vi "GPS-1仪器串口通讯.vi"(0 "VISA resource name":refnum<visa-resource-name>="COM3", 4 "baud rate (9600)":u32=9600, 7 "错误常量 2":errorcluster caption="错误常量") -> (11 "错误常量":errorcluster, 12 "速率":string, 13 "经度":string, 14 "定位信息":string, 15 "UTC日期":string, 17 "航向":string, 18 "UTC时间":string, 19 "纬度":string)   [LabVIEW 2016]
uses:
  <vilib>/Instr/_visa.llb/VISA Configure Serial Port (Instr).vi
panel:
  out "数组":string[](array[string])
  out "字符串 3":string
  out "长度 2":i32
  in  "字符串 2":string
  out "长度":i32
  in  "字符串":string
  out "返回数 2":u32
  out "read buffer":string
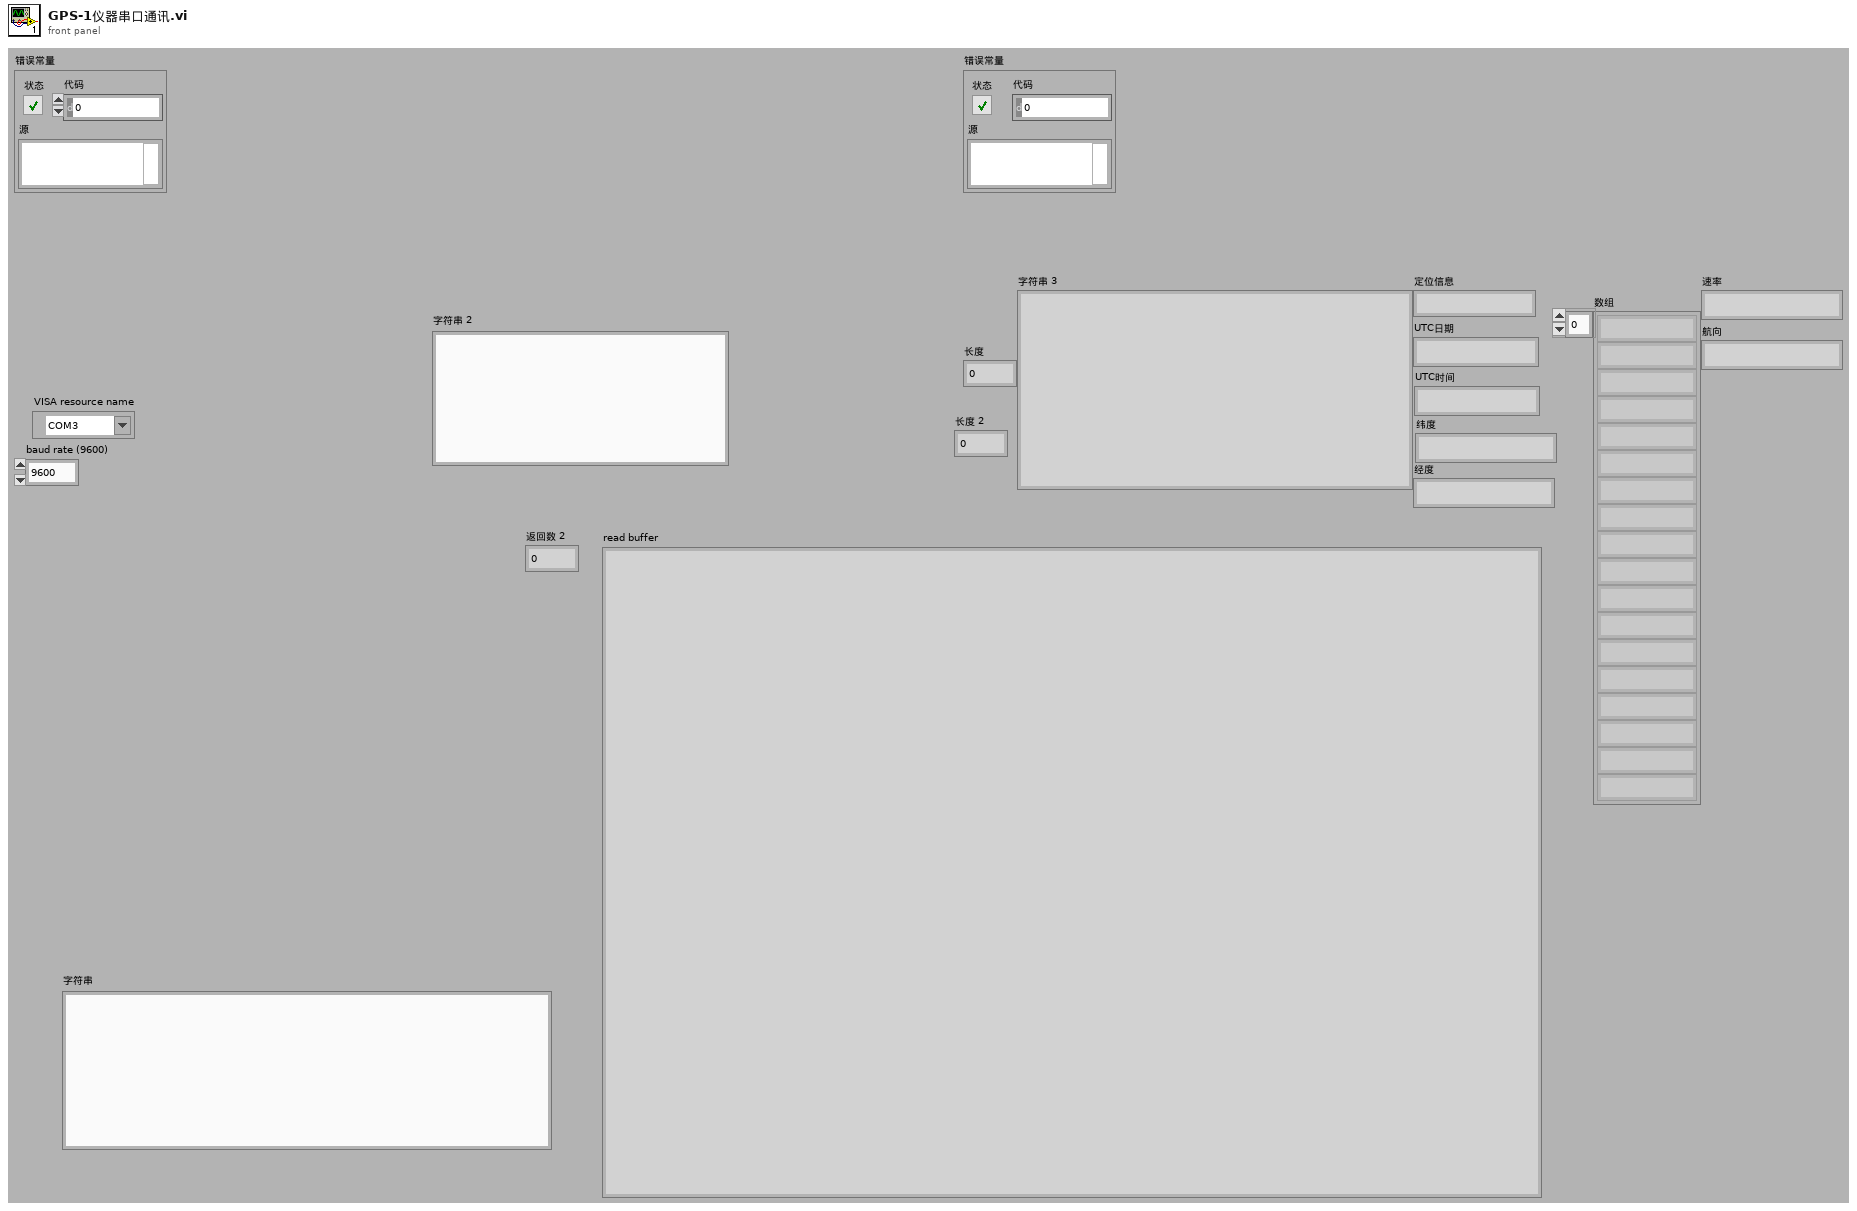
[diagram p1: front panel]
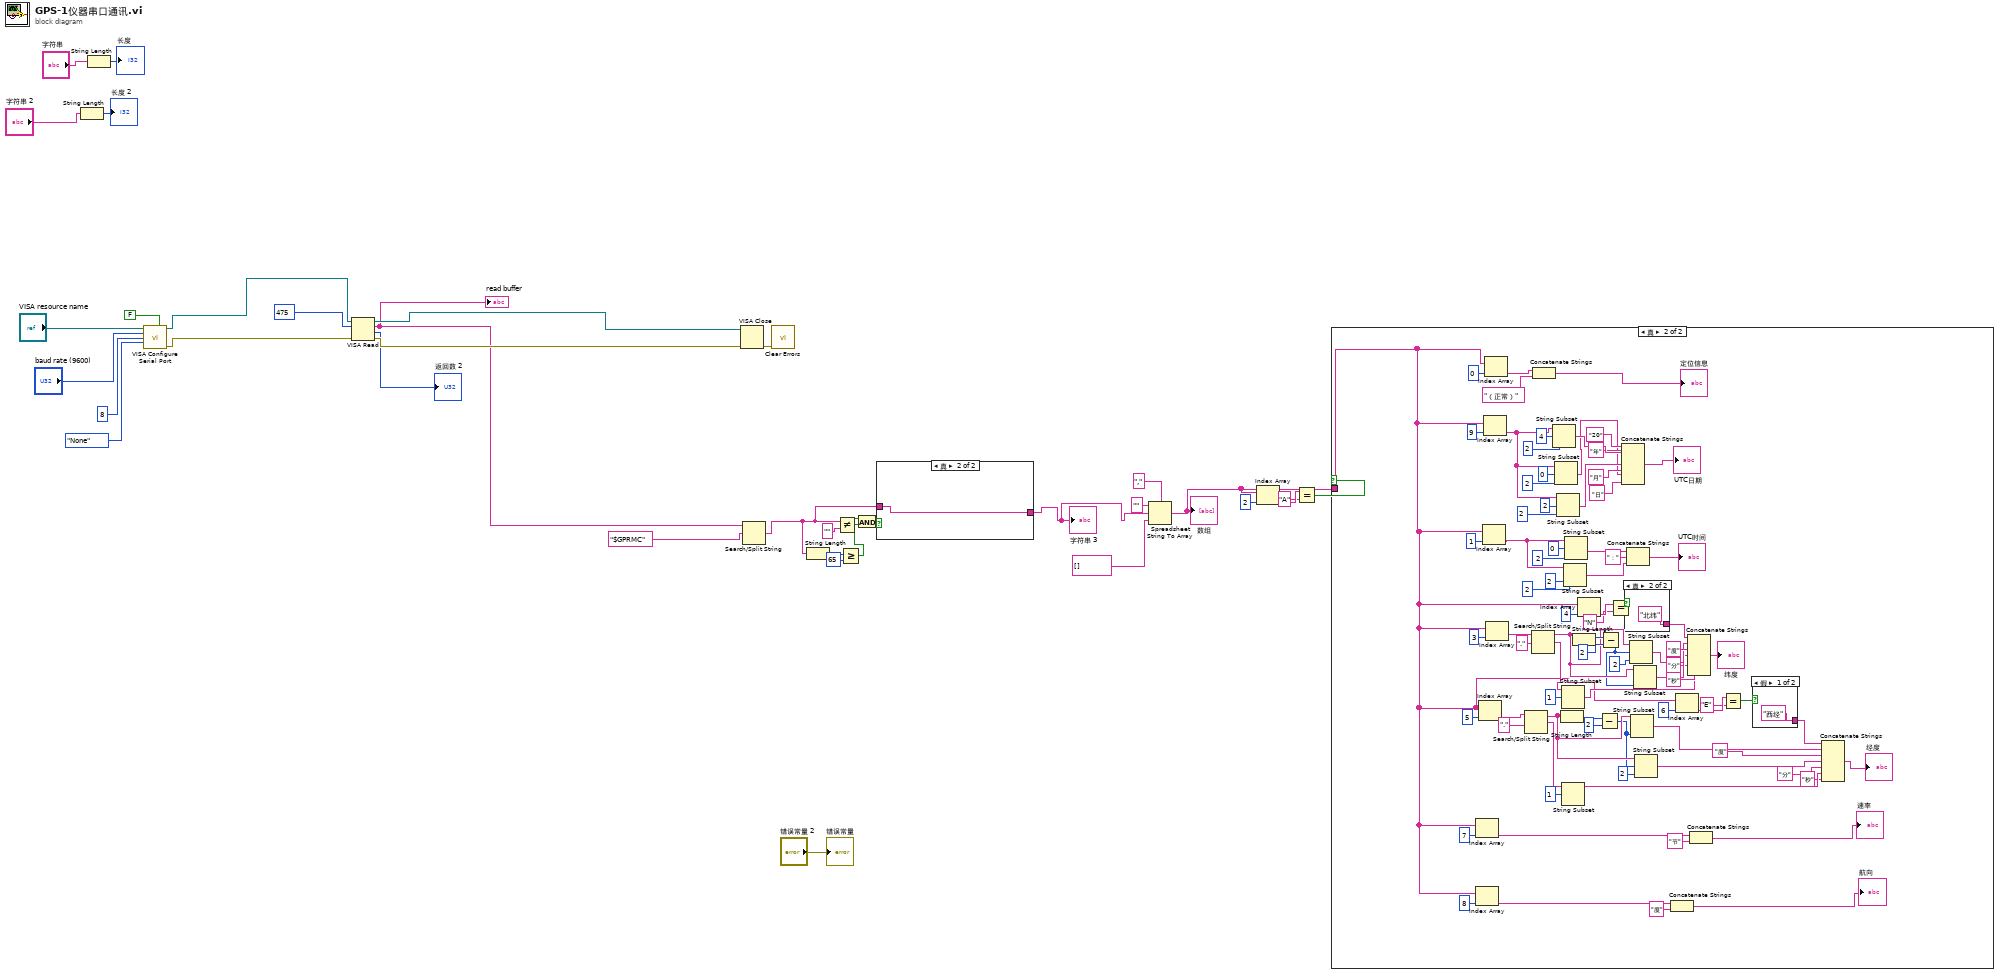
[diagram p0: block diagram]
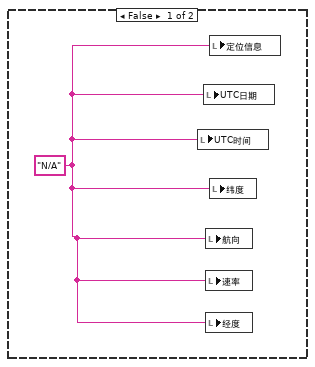
[diagram p2: hidden frame]
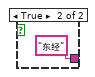
[diagram p3: hidden frame]
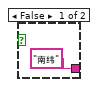
[diagram p4: hidden frame]
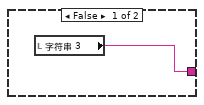
[diagram p5: hidden frame]
diagram:
  n1 = String Length(string="字符串 2") -> (length=→"长度 2":i32)
  n2 = String Length(string="字符串") -> (length=→"长度":i32)
  n3 = call-poly "VISA Configure Serial Port"("VISA resource name"="VISA resource name", "Enable Termination\nChar (T)"=FALSE ("Enable Termination\nChar (T)"), "baud rate (9600)"="baud rate (9600)", "data bits (8)"=u16 8, "parity (0:none)"=enum16{"None", "Odd", "Even", "Mark", "Space"}."None") -> ("VISA resource name out"=w23:refnum<visa-resource-name>, "error out"=w27:errorcluster)  [unwired: 9 in]
  n4 = VISA Read(VISA resource name=w23, byte count=u32 475 ("字节总数"), error in (no error)=w27) -> (VISA resource name out=w26:refnum<visa-resource-name>, read buffer=w19:string, return count=→"返回数 2":u32, error out=w32:errorcluster)
  "read buffer" <- w19
  n5 = VISA Close(VISA resource name=w26, error in (no error)=w32) -> (error out=w29:errorcluster)
  n6 = Search/Split String(string=w19, search string/char (-)="$GPRMC" ("搜索字符串/字符(-)")) -> (match + rest of string=w13:string)  [unwired: 1 in, 2 out]
  n7 = call <vilib>:"Clear Errors.vi"("error in (no error)"=w29) -> ()  [unwired: 5 in, 2 out]
  n8 = String Length(string=w13) -> (length=w14:i32)
  n9 = Not Equal?(x=w13, y="") -> (x != y?=w16:bool)
  n10 = Greater Or Equal?(x=w14, y=65) -> (x >= y?=w11:bool)
  n11 = And(x=w11, y=w16) -> (x .and. y?=w15:bool)
  n12 = case shown="真" w15 {
    tunnel: w13 -> [_ w37]
    tunnel: [w36 w37] -> w10
    frame False {
      n13 = local read "字符串 3"() -> (w36:string)
    }
    frame True {
    }
  }
  "字符串 3" <- w10
  n14 = Spreadsheet String To Array(delimiter (Tab)="," ("分隔符(Tab)"), format string="" ("格式字符串"), spreadsheet string=w10, array type (2D Dbl)=string[] []) -> (array=w6:string[])
  "数组" <- w6
  n15 = Index Array(array=w6, index=2 ("索引")) -> (element=w4:string)
  n16 = Equal?(x=w4, y="A") -> (x = y?=w2:bool)
  n17 = case shown="真" w2 {
    tunnel: w6 -> [_ w48]
    frame False {
      w38 = "N/A"
      n18 = local write "UTC时间"(w38) -> ()
      n19 = local write "UTC日期"(w38) -> ()
      n20 = local write "航向"(w38) -> ()
      n21 = local write "速率"(w38) -> ()
      n22 = local write "经度"(w38) -> ()
      n23 = local write "定位信息"(w38) -> ()
      n24 = local write "纬度"(w38) -> ()
    }
    frame True {
      n25 = Index Array(array=w48, index=7 ("索引")) -> (element=w46:string)
      n26 = Index Array(array=w48, index=8 ("索引")) -> (element=w45:string)
      n27 = Index Array(array=w48, index=5 ("索引")) -> (element=w70:string)
      n28 = Index Array(array=w48, index=1 ("索引")) -> (element=w98:string)
      n29 = Index Array(array=w48, index=9 ("索引")) -> (element=w109:string)
      n30 = Index Array(array=w48, index=0 ("索引")) -> (element=w120:string)
      n31 = Index Array(array=w48, index=3 ("索引")) -> (element=w86:string)
      n32 = Search/Split String(string=w70, search string/char (-)="." ("搜索字符串/字符(-)")) -> (substring before match=w59:string, match + rest of string=w54:string)  [unwired: 1 in, 1 out]
      n33 = Search/Split String(string=w86, search string/char (-)="." ("搜索字符串/字符(-)")) -> (substring before match=w81:string, match + rest of string=w74:string)  [unwired: 1 in, 1 out]
      n34 = Concatenate Strings(w120, "（正常）" ("字符串")) -> (→"定位信息":string)
      n35 = String Subset(string=w109, offset (0)=4 ("偏移量(0)"), length (rest)=2 ("长度（剩余）")) -> (substring=w111:string)
      n36 = String Subset(string=w109, offset (0)=0 ("偏移量(0)"), length (rest)=2 ("长度（剩余）")) -> (substring=w39:string)
      n37 = String Subset(string=w109, offset (0)=2 ("偏移量(0)"), length (rest)=2 ("长度（剩余）")) -> (substring=w40:string)
      n38 = String Length(string=w59) -> (length=w68:i32)
      n39 = String Subset(string=w74, offset (0)=1 ("偏移量(0)")) -> (substring=w72:string)  [unwired: 1 in]
      n40 = String Subset(string=w54, offset (0)=1 ("偏移量(0)")) -> (substring=w53:string)  [unwired: 1 in]
      n41 = String Subset(string=w98, offset (0)=2 ("偏移量(0)"), length (rest)=2 ("长度（剩余）")) -> (substring=w95:string)
      n42 = String Subset(string=w98, offset (0)=0 ("偏移量(0)"), length (rest)=2 ("长度（剩余）")) -> (substring=w97:string)
      n43 = String Length(string=w81) -> (length=w83:i32)
      n44 = Index Array(array=w48, index=4 ("索引")) -> (element=w90:string)
      n45 = Subtract(x=w68, y=2) -> (x-y=w58:i32)
      n46 = Subtract(x=w83, y=2) -> (x-y=w80:i32)
      n47 = Equal?(x=w90, y="N") -> (x = y?=w88:bool)
      n48 = Concatenate Strings("20" ("字符串"), w111, "年" ("字符串"), w40, "月" ("字符串"), w39, "日" ("字符串")) -> (→"UTC日期":string)
      n49 = case shown="真" w88 {
        tunnel: ["南纬" ("字符串") "北纬" ("字符串")] -> w91
        frame False {
        }
        frame True {
        }
      }
      n50 = Concatenate Strings(w97, "：" ("字符串"), w95) -> (→"UTC时间":string)
      n51 = String Subset(string=w81, offset (0)=w80, length (rest)=2 ("长度（剩余）")) -> (substring=w78:string)
      n52 = String Subset(string=w59, length (rest)=w58) -> (substring=w66:string)  [unwired: 1 in]
      n53 = String Subset(string=w81, length (rest)=w80) -> (substring=w79:string)  [unwired: 1 in]
      n54 = String Subset(string=w59, offset (0)=w58, length (rest)=2 ("长度（剩余）")) -> (substring=w56:string)
      n55 = Concatenate Strings(w45, "度" ("字符串")) -> (→"航向":string)
      n56 = Index Array(array=w48, index=6 ("索引")) -> (element=w63:string)
      n57 = Concatenate Strings(w91, w79, "度" ("字符串"), w78, "分" ("字符串"), w72, "秒" ("字符串")) -> (→"纬度":string)
      n58 = Concatenate Strings(w46, "节" ("字符串")) -> (→"速率":string)
      n59 = Equal?(x=w63, y="E") -> (x = y?=w61:bool)
      n60 = case shown="假" w61 {
        tunnel: ["西经" ("字符串") "东经" ("字符串")] -> w60
        frame False {
        }
        frame True {
        }
      }
      n61 = Concatenate Strings(w60, w66, "度" ("字符串"), w56, "分" ("字符串"), w53, "秒" ("字符串")) -> (→"经度":string)
    }
  }
  "错误常量" <- "错误常量 2"
